vi "Report Generator.vi"(8 "error in (no error)":errorcluster, 11 "Report Generator In":refnum<class "Report Generator.lvclass">) -> (0 "error out":errorcluster)   [LabVIEW 2020, in "Report Generation.lvlib" / "Report Generator.lvclass"]
uses:
  Report Generator.lvclass
  C:/git/astemes-lunit/source/User Interface/Process/Process.lvclass
  User Interface/Process/Process.lvclass/Process.ctl
  Report Generator.lvclass/Report Generator.ctl
  Report Interface/Report Interface.lvclass
  User Interface/Process/Process.lvclass
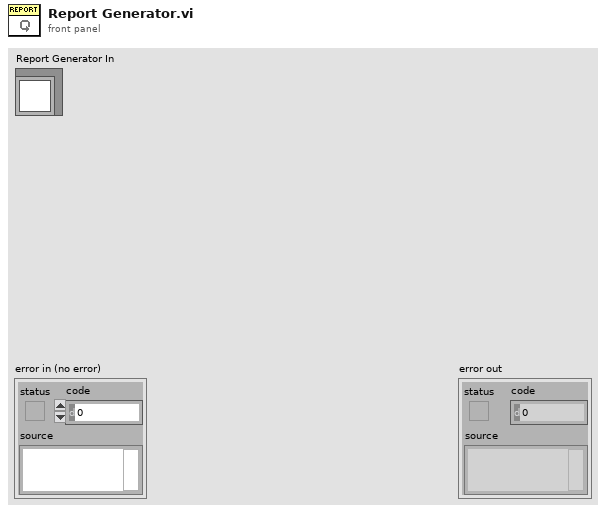
[diagram p1: front panel]
types:
  T1 = typedef "Result.lvlib/Result.ctl" = cluster{"Name":string, "Description":string, "Status":T2, "Result Type":T3, "Execution Time":dbl, "Data":cluster{"Expected":variant, "Actual":variant, "Delta":variant}}
  T2 = typedef "Result.lvlib/Status.ctl" = enum16{"", "Passed", "Failed", "Error", "Skipped", "Setup Error", "Broken", "Teardown Error"}
  T3 = typedef "Result.lvlib/Type.ctl" = enum16{"Test Case", "Test Suite", "Test Run", "Pass", "Fail", "Skip", "Pass if", "Fail if", "Pass if Error", "Fail if Error", "Pass if Equal", "Fail if Equal"}
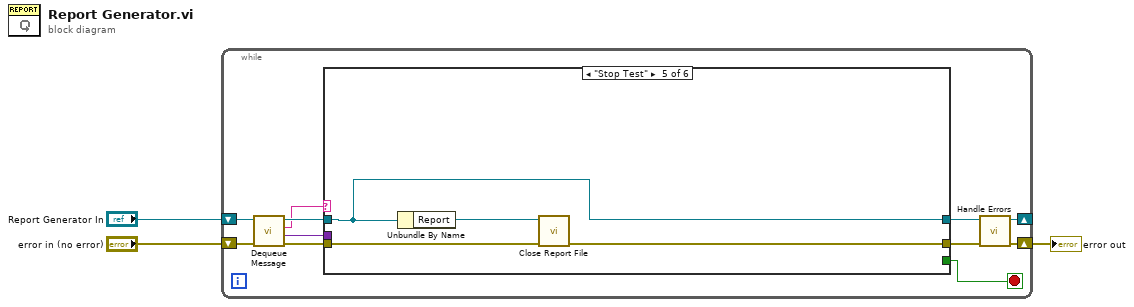
[diagram p0: block diagram]
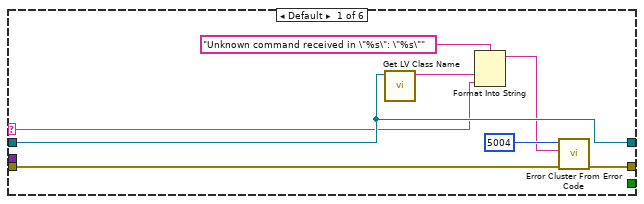
[diagram p2: hidden frame]
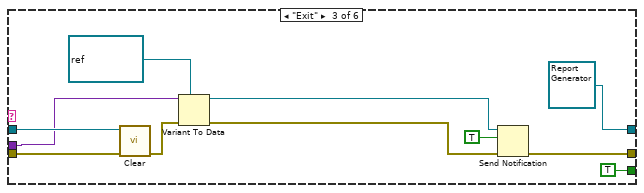
[diagram p4: hidden frame]
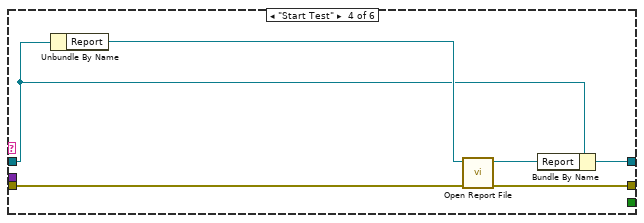
[diagram p5: hidden frame]
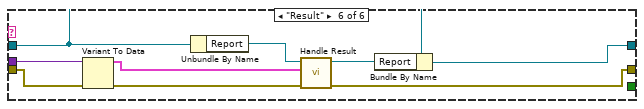
[diagram p6: hidden frame]
diagram:
  n1 = while {
    shift-right: [w6] -> w1
    shift-left: "error in (no error)" -> [w13]
    shift-right: [w8] -> _
    shift-left: "Report Generator In" -> [w11]
    stop <- w7 stop-if-true
    n2 = call "Dequeue Message.vi"("error in (no error)"=w13, "Process In"=w11) -> ("error out"=w12:errorcluster, "Message Data"=w10:variant, "Message"=w5:string, "Process Out"=w9:refnum<class "Report Generator.lvclass">)  [unwired: 6 in]
    n3 = case shown="\"Stop Test\"" w5 {
      selector: w5 -> [w18 _ _ _ _ _]
      tunnel: w12 -> [w21 w22 w32 w35 w44 w53]
      tunnel: [w20 w22 w30 w40 w43 w52] -> w4
      tunnel: w10 -> [_ _ w29 _ _ w50]
      tunnel: w9 -> [w19 w23 w33 w36 w41 w46]
      tunnel: [w19 w23 refnum<class "Report Generator.lvclass"> refnum ("Process Out") w38 w41 w47] -> w8
      tunnel: [_ _ TRUE _ _ _] -> w7
      frame Default {
        n4 = call <vilib>:"Get LV Class Name.vi"("object"=w19) -> ("class name"=w17:string)  [unwired: 9 in, 1 out]
        n5 = Format Into String(format string="Unknown command received in \"%s\": \"%s\"", w17, w18) -> (resulting string=w14:string)  [unwired: 2 in, 1 out]
        n6 = call <vilib>:"Error Cluster From Error Code.vi"("error in (no error)"=w21, "error message (\"\")"=w14, "error code (0)"=5004) -> ("error out"=w20:errorcluster)  [unwired: 6 in]
      }
      frame "Init" {
      }
      frame "Exit" {
        n7 = call-dynamic "Clear.vi"("error in (no error)"=w32, "Process In"=w33) -> ("error out"=w27:errorcluster)  [unwired: 9 in]
        n8 = Variant To Data(error in=w27, type=refnum<notifier> refnum ("notifier out"), Variant=w29) -> (data=w25:refnum<notifier>, error out=w26:errorcluster)
        n9 = Send Notification(notification=TRUE, notifier=w25, error in (no error)=w26) -> (error out=w30:errorcluster)  [unwired: 1 out]
      }
      frame "Start Test" {
        n10 = Unbundle By Name(w36) -> ("Report"=w39:refnum<class "Report Interface.lvclass">)
        n11 = call-dynamic "Open Report File.vi"("error in (no error)"=w35, "Report Interface In"=w39) -> ("error out"=w40:errorcluster, "Report Interface Out"=w37:refnum<class "Report Interface.lvclass">)  [unwired: 8 in]
        n12 = Bundle By Name(cluster=w36, "Report"=w37) -> (w38:refnum<class "Report Generator.lvclass">)
      }
      frame "Stop Test" {
        n13 = Unbundle By Name(w41) -> ("Report"=w42:refnum<class "Report Interface.lvclass">)
        n14 = call-dynamic "Close Report File.vi"("error in (no error)"=w44, "Report Interface In"=w42) -> ("error out"=w43:errorcluster)  [unwired: 8 in, 1 out]
      }
      frame "Result" {
        n15 = Variant To Data(error in=w53, Variant=w50) -> (data=w49:T1, error out=w51:errorcluster)  [unwired: 1 in]
        n16 = Unbundle By Name(w46) -> ("Report"=w48:refnum<class "Report Interface.lvclass">)
        n17 = call-dynamic "Handle Result.vi"("error in (no error)"=w51, "Result"=w49, "Report in"=w48) -> ("error out"=w52:errorcluster, "Report out"=w45:refnum<class "Report Interface.lvclass">)  [unwired: 7 in]
        n18 = Bundle By Name(cluster=w46, "Report"=w45) -> (w47:refnum<class "Report Generator.lvclass">)
      }
    }
    n19 = call "Handle Errors.vi"("error in (no error)"=w4) -> ("error out"=w6:errorcluster)  [unwired: 10 in]
  }
  "error out" <- w1
